vi "Analog to Serial Port.vi"   [LabVIEW 2014]
uses:
  <vilib>/Aledyne-TSXperts/Arduino Compatible Compiler for LabVIEW/Arduino Compatible Compiler for LabVIEW.lvlib
  QwaveSys_ESP8266/QwaveSys_ESP8266.lvlib
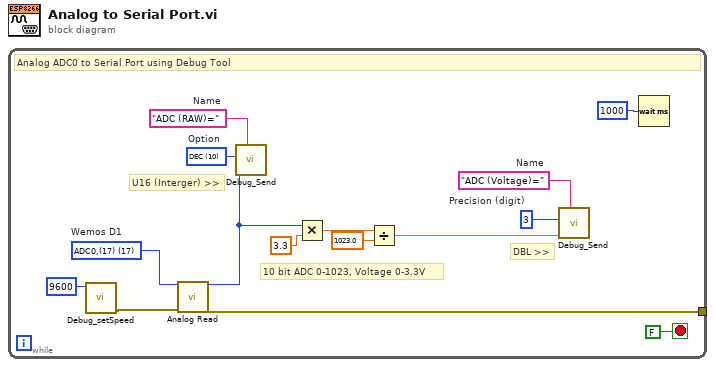
[diagram p0: block diagram]
diagram:
  n1 = while {
    tunnel: [w8] -> _
    stop <- FALSE stop-if-true
    w1 = u16 10 items=["DEC"=10, "HEX"=16, "OCT"=8, "BIN"=2]  # Option
    w3 = "ADC (RAW)="  # Name
    w4 = 3  # Precision (digit)
    w5 = "ADC (Voltage)="  # Name
    w7 = u8 17 items=["D0-RX(3)"=3, "D1-TX(1)"=1, "D2(16)"=16, "D3/D15/SCL(5)"=5, "D4/D14/SDA(4)"=4, "D5/D13/SCK(14)-(LED)"=14, "D6/D12/MISO(12)"=12, "D7/D11/MOSI(13)"=13, "D8(0)"=0, "D9/TX1(2)"=2, "D10/SS (15)"=15, "ADC0,(17)"=17]  # Wemos D1
    # "U16 (Interger) >>"
    # "DBL >>"
    # "10 bit ADC 0-1023, Voltage 0-3.3V"
    # "Analog ADC0 to Serial Port using Debug Tool"
    n2 = call "Debug_setSpeed.vi"("Speed"=u32 9600) -> ("error out"=w9:errorcluster)  [unwired: 10 in]
    n3 = call <vilib>:"Analog Read.vi"("pin"=w7, "error in (no error)"=w9) -> ("data"=w2:u16, "error out"=w8:errorcluster)  [unwired: 12 in]
    n4 = call "Debug_Send.vi"("Name"=w3, "DATA"=w2, "Option"=w1) -> ()  [unwired: 9 in]
    n5 = Multiply(x=w2, y=3.3) -> (x*y=w12:dbl)
    n6 = Divide(x=w12, y=1023.0 ("x")) -> (x/y=w6:dbl)
    n7 = call "Debug_Send.vi"("Name"=w5, "DATA"=w6, "Option"=w4) -> ()  [unwired: 9 in]
    n8 = Wait (ms)(milliseconds to wait=u32 1000) -> ()  [unwired: 1 out]
  }
